vi "Recieve Status.vi"(6 "bytes to read":i32=4, 8 "error in (no error)":errorcluster, 9 "Status offset":u64, 10 "Read config instead":bool, 11 "RP Communicator in":refnum<class "RP Communicator.lvclass">) -> (0 "error out":errorcluster, 1 "Status response":u32=1 format="0x%x (%d)", 3 "RP Communicator out":refnum<class "RP Communicator.lvclass">)   [LabVIEW 2024, in "RP Communicator.lvclass"]
uses:
  RP Communicator.lvclass
  RP Communicator.lvclass/RP Communicator.ctl
  RP Read Status TCP.vi
panel:
  in  "Calls":i64
  out "attempts":i32
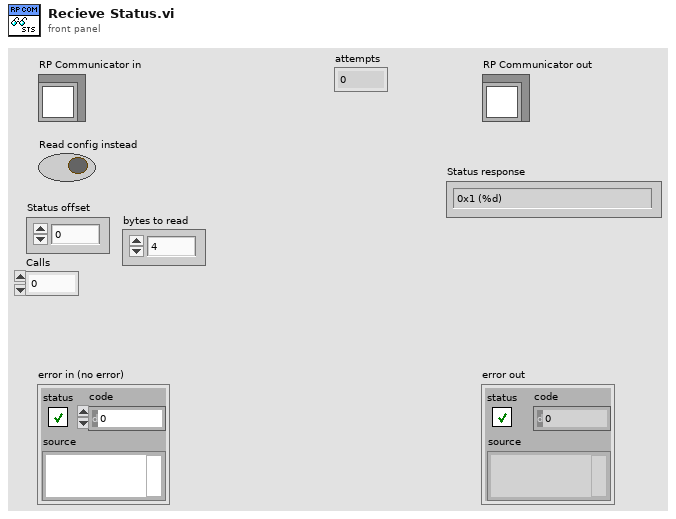
[diagram p1: front panel]
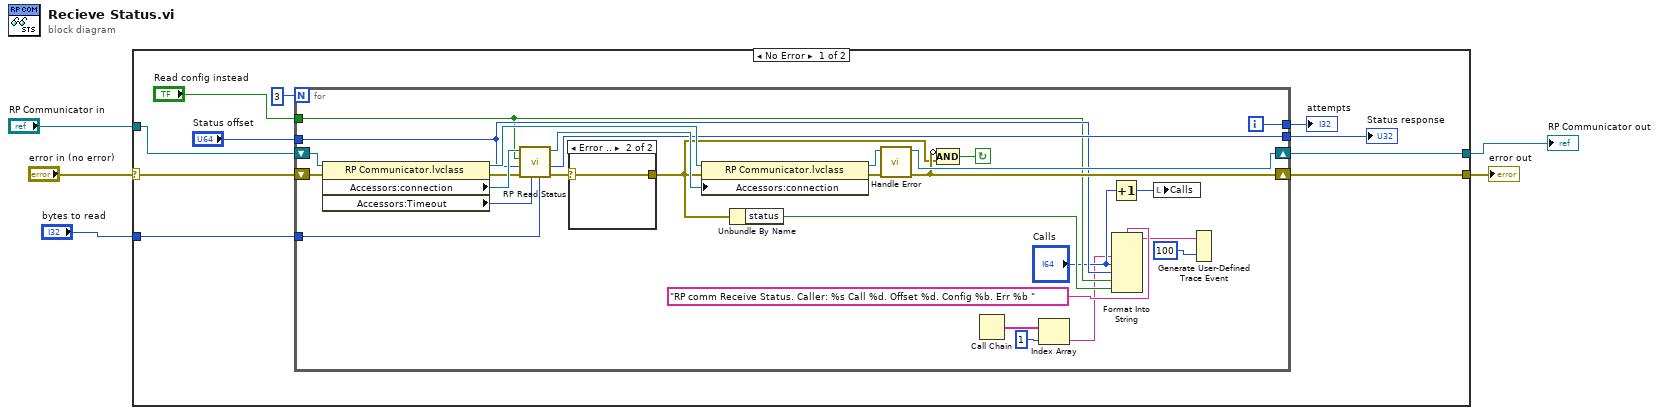
[diagram p0: block diagram]
diagram:
  n1 = case shown="No Error" "error in (no error)" {
    selector: "error in (no error)" -> [w12 w47]
    tunnel: [w13 w47] -> w4
    tunnel: [w14 w46] -> w2
    tunnel: "RP Communicator in" -> [w15 w46]
    tunnel: "bytes to read" -> [w6 _]
    frame No Error {
      n2 = for {
        N: 3 -> [_]
        tunnel: "Status offset" -> [w25]
        tunnel: "Read config instead" -> [w24]
        tunnel: [w36] -> w9
        shift-right: [w32] -> w14
        shift-left: w15 -> [w43]
        shift-right: [w30] -> w13
        shift-left: w12 -> [w38]
        tunnel: [w35] -> w7
        tunnel: w6 -> [w16]
        i -> [w35]
        stop <- w31 continue-if-true
        n3 = property class="RP Communicator.lvclass"(reference=w43, error in=w38) -> (reference out=w42:refnum<class "RP Communicator.lvclass">, error out=w39:errorcluster, "Accessors:connection"=w41:refnum<k5>, "Accessors:Timeout"=w37:i32)
        n4 = call-poly "RP Read Status.vi"("bytes to read"=w16, "timeout ms (25000)"=w37, "Error In"=w39, "Status offset"=w25, "Read config"=w24, "connection ID"=w41) -> ("Error Out"=w18:errorcluster, "Status response"=w36:u32, "connection ID out"=w40:refnum<k5>)  [unwired: 3 in]
        n5 = case shown="Error .." w18 {
          selector: w18 -> [w44 w45]
          tunnel: [w44 w45] -> w17
          frame No Error {
          }
          frame Error {
          }
        }
        n6 = property class="RP Communicator.lvclass"(reference=w42, error in=w17, "Accessors:connection"=w40) -> (reference out=w33:refnum<class "RP Communicator.lvclass">, error out=w34:errorcluster)
        n7 = Unbundle By Name(w17) -> ("status"=w23:bool)
        n8 = call-dynamic "Handle Error.vi"("error in (no error)"=w34, "RP Communicator in"=w33) -> ("error out"=w30:errorcluster, "RP Communicator out"=w32:refnum<class "RP Communicator.lvclass">)  [unwired: 8 in]
        n9 = Compound Arithmetic op=AND(invert w30, w17) -> (w31:bool)
        n10 = Call Chain() -> (call chain=w22:string[])
        n11 = Index Array(array=w22, index=1) -> (element=w19:string)
        n12 = Increment(x="Calls") -> (x+1=w26:i64)
        n13 = Format Into String(format string="RP comm Receive Status. Caller: %s Call %d. Offset %d. Config %b. Err %b ", w19, "Calls", w25, w24, w23) -> (resulting string=w27:string)  [unwired: 2 in, 1 out]
        n14 = local write "Calls"(w26) -> ()
        n15 = Generate User-Defined Trace Event(1:100 ("trace integer"), 2:w27) -> ()
      }
      "Status response" <- w9
      "attempts" <- w7
    }
    frame Error {
    }
  }
  "error out" <- w4
  "RP Communicator out" <- w2
